vi "SIM Registry Register Node (scalar).vi"(4 "Tag":string, 10 "Has ZC?":bool, 11 "Registry In":T1) -> (2 "Block Idx":i32, 3 "Registry Out":T1)   [LabVIEW 2017]
uses:
  <vilib>/Simulation/Implementation/Shared/SIM Registry.llb/SIM Simulation Registry.ctl
  <vilib>/Simulation/Implementation/Shared/SIM Registry.llb/SIM Registry Node Header.ctl
  <vilib>/Simulation/Implementation/Shared/SIM Registry.llb/SIM Registry Node Record.ctl
  <vilib>/Simulation/Implementation/Shared/SIM trigger type.ctl
  <vilib>/Simulation/Implementation/Shared/SIM solver state data.ctl
  <vilib>/Simulation/Implementation/Shared/SIM limit type.ctl
  <vilib>/Simulation/Implementation/Shared/SIM discrete data.ctl
  <vilib>/Simulation/Implementation/Shared/SIM Discrete state data.ctl
  <vilib>/Simulation/Implementation/Shared/SIM Registry.llb/SIM Simulation Registry Error.ctl
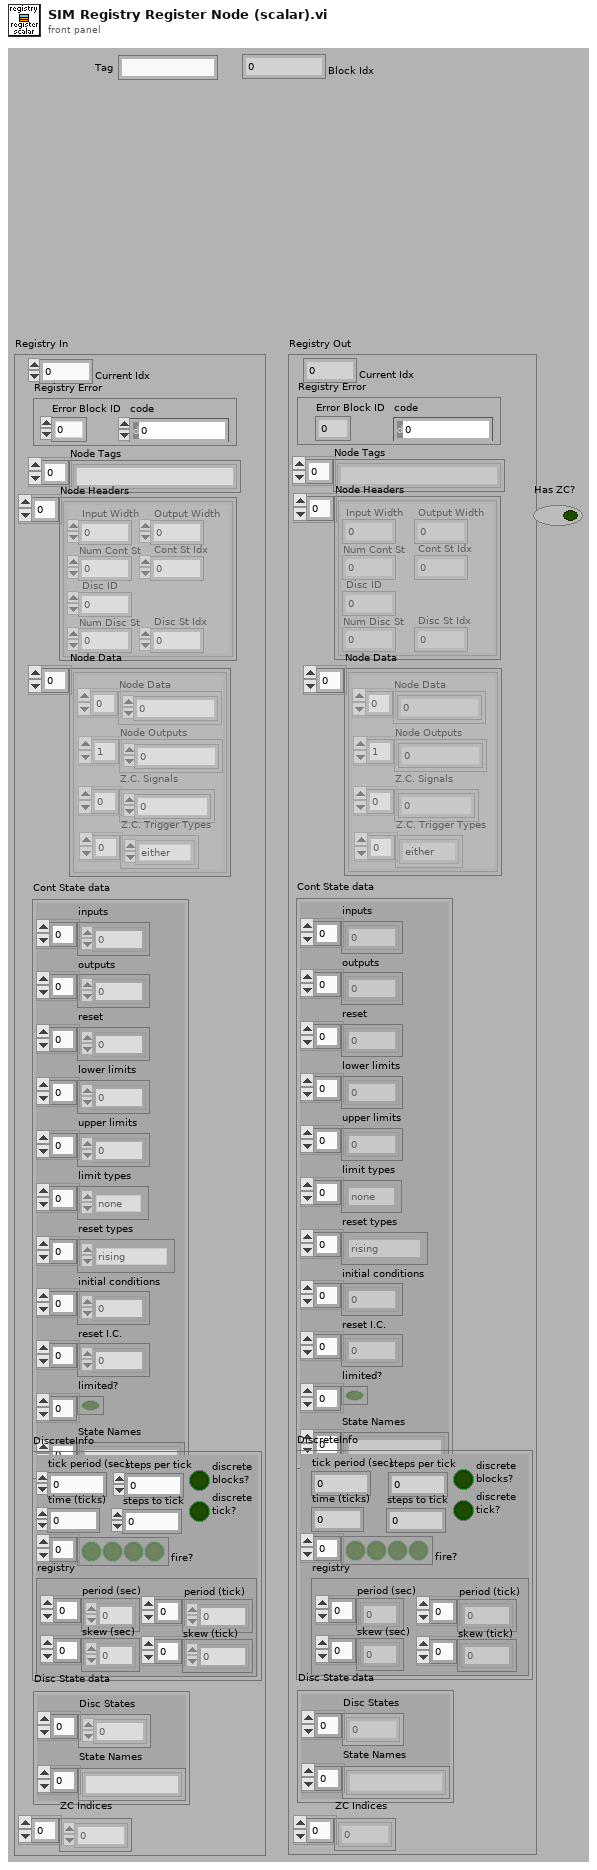
[diagram p1: front panel]
types:
  T1 = typedef "SIM Simulation Registry.ctl" = cluster{"Current Idx":i32, "Node Tags":string[], "Node Headers":T2[], "Node Data":T3[], "Cont State data":T5, "DiscreteInfo":T7, "Disc State data":T8, "Registry Error":T9, "ZC Indices":i32[]}
  T2 = typedef "SIM Registry Node Header.ctl" = cluster{"Input Width":i32, "Disc ID":i32, "Num Cont St":i32, "Cont St Idx":i32, "Num Disc St":i32, "Disc St Idx":i32, "Output Width":i32}
  T3 = typedef "SIM Registry Node Record.ctl" = cluster{"Node Data":dbl[], "Node Outputs":dbl[], "Z.C. Signals":dbl[], "Z.C. Trigger Types":T4[]}
  T4 = typedef "SIM trigger type.ctl" = enum16{"rising", "falling", "either", "none"}
  T5 = typedef "SIM solver state data.ctl" = cluster{"inputs":dbl[], "outputs":dbl[], "reset":dbl[], "lower limits":dbl[], "upper limits":dbl[], "limit types":T6[], "reset types":T4[], "initial conditions":dbl[], "reset I.C.":dbl[], "limited?":bool[], "State Names":string[]}
  T6 = typedef "SIM limit type.ctl" = enum16{"upper", "lower", "both", "none"}
  T7 = typedef "SIM discrete data.ctl" = cluster{"tick period (sec)":dbl, "time (ticks)":i32, "fire?":bool[], "registry":cluster{"period (sec)":dbl[], "skew (sec)":dbl[], "period (tick)":i32[], "skew (tick)":i32[]}, "discrete \nblocks?":bool, "steps per tick":dbl, "steps to tick":dbl, "discrete \ntick?":bool}
  T8 = typedef "SIM Discrete state data.ctl" = cluster{"Disc States":dbl[], "State Names":string[]}
  T9 = typedef "SIM Simulation Registry Error.ctl" = cluster{"Error Block ID":i32, "code":i32}
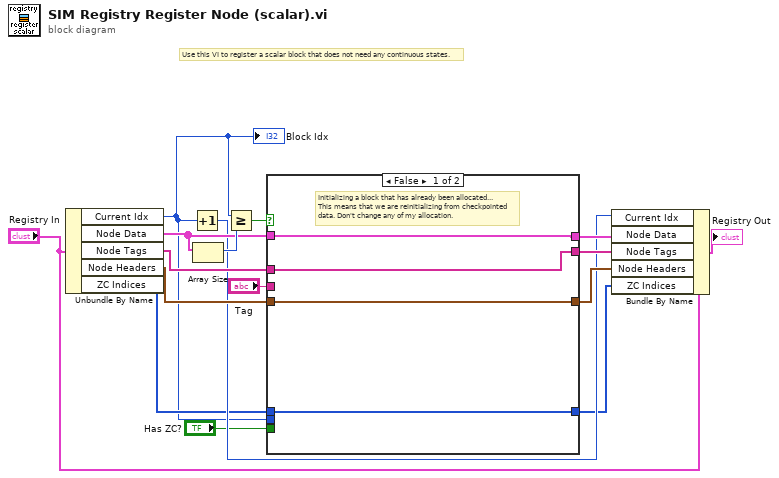
[diagram p0: block diagram]
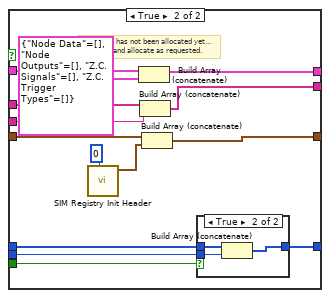
[diagram p2: hidden frame]
diagram:
  # "Use this VI to register a scalar block that does not need any continuous states."
  n1 = Unbundle By Name("Registry In") -> ("Current Idx"=w2:i32, "Node Data"=w14:T3[], "Node Tags"=w9:string[], "Node Headers"=w7:T2[], "ZC Indices"=w4:i32[])
  "Block Idx" <- w2
  n2 = Increment(x=w2) -> (x+1=w5:i32)
  n3 = Array Size(array=w14) -> (size(s)=w16:i32)
  n4 = Greater Or Equal?(x=w2, y=w16) -> (x >= y?=w15:bool)
  n5 = case shown="False" w15 {
    tunnel: w14 -> [w20 w33]
    tunnel: "Tag" -> [_ w30]
    tunnel: [w20 w32] -> w10
    tunnel: w9 -> [w19 w31]
    tunnel: [w19 w29] -> w8
    tunnel: w7 -> [w18 w27]
    tunnel: [w18 w25] -> w6
    tunnel: w4 -> [w17 w24]
    tunnel: "Has ZC?" -> [_ w23]
    tunnel: w2 -> [_ w22]
    tunnel: [w17 w21] -> w1
    frame False {
      # "Initializing a block that has already been allocated...\nThis means that we are reinitializing from checkpointed\ndata. Don't change any of my allocation."
    }
    frame True {
      # "This block has not been allocated yet...\nGo ahead and allocate as requested."
      n6 = call <vilib>:"SIM Registry Init Header.vi"("Input Width"=0 ("Signal Width")) -> ("Node Header"=w26:T2)  [unwired: 7 in, 3 out]
      n7 = Build Array (concatenate)(w33, T3 {"Node Data"=[], "Node Outputs"=[], "Z.C. Signals"=[], "Z.C. Trigger Types"=[]} ("Node Record")) -> (w32:T3[])
      n8 = Build Array (concatenate)(w31, w30) -> (w29:string[])
      n9 = Build Array (concatenate)(w27, w26) -> (w25:T2[])
      n10 = case shown="True" w23 {
        tunnel: w22 -> [_ w37]
        tunnel: w24 -> [w35 w38]
        tunnel: [w35 w36] -> w21
        frame False {
        }
        frame True {
          n11 = Build Array (concatenate)(w38, w37) -> (w36:i32[])
        }
      }
    }
  }
  n12 = Bundle By Name(cluster="Registry In", "Current Idx"=w5, "Node Data"=w10, "Node Tags"=w8, "Node Headers"=w6, "ZC Indices"=w1) -> (→"Registry Out":T1)
